vi "Receive Message.vi"(8 "error in (no error)":errorcluster, 10 "Message":refnum<class "Message.lvclass">, 11 "Actor in":refnum<class "Actor.lvclass">) -> (0 "error out":errorcluster, 2 "Stop Actor":bool, 3 "Actor out":refnum<class "Actor.lvclass">)   [LabVIEW 2020, in "Artifex.lvlib" / "Actor.lvclass"]
uses:
  Actor.lvclass
  Message/Message.lvclass
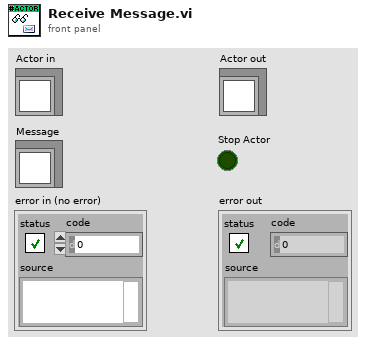
[diagram p1: front panel]
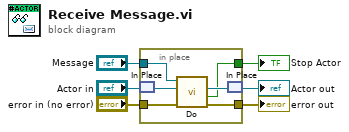
[diagram p0: block diagram]
diagram:
  n1 = in-place {
    in-place-border: "error in (no error)" -> [w12]
    in-place-border: [w11] -> w5
    in-place-border: "Message" -> [w10]
    in-place-border: [w7] -> w1
    n2 = in-place-match #1("Actor in") -> (w9:refnum<class "Actor.lvclass">)
    n3 = call-dynamic "Do.vi"("error in (no error)"=w12, "Actor In"=w9, "Message in"=w10) -> ("error out"=w11:errorcluster, "Stop Actor"=w7:bool, "Actor Out"=w8:refnum<class "Actor.lvclass">)  [unwired: 6 in]
    n4 = in-place-match #1(w8) -> (→"Actor out":refnum<class "Actor.lvclass">)
  }
  "error out" <- w5
  "Stop Actor" <- w1
